vi "GetObserverList.vi"(8 "error in (no error)":errorcluster, 11 "Observable in":refnum<class "Observable.lvclass">) -> (0 "error out":errorcluster, 2 "ObserverClassName":string[](array[string]), 3 "Observable out":refnum<class "Observable.lvclass">)   [LabVIEW 2013, in "Observable.lvclass"]
uses:
  Observable.lvclass
  Observable.lvclass/Observable.ctl
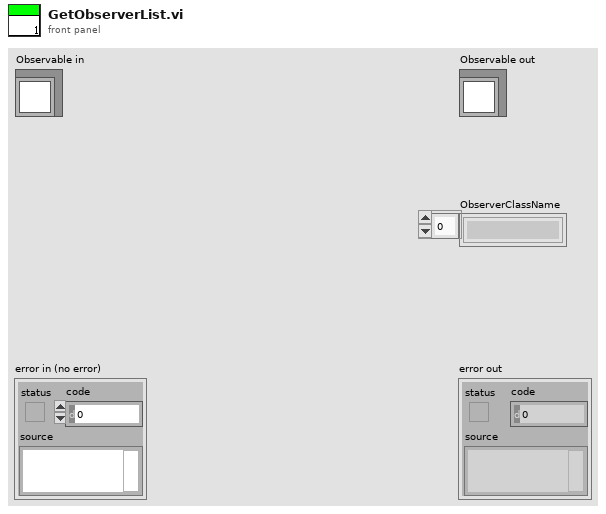
[diagram p1: front panel]
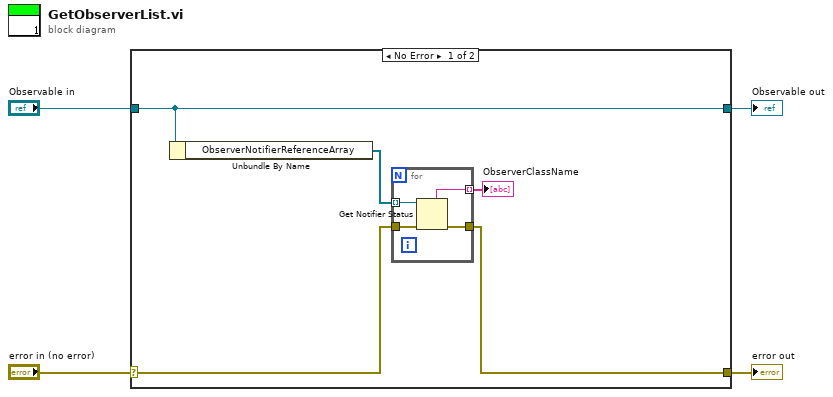
[diagram p0: block diagram]
diagram:
  n1 = case shown="No Error" "error in (no error)" {
    selector: "error in (no error)" -> [w7 w15]
    tunnel: [w6 w15] -> w3
    tunnel: [w9 w14] -> w1
    tunnel: "Observable in" -> [w9 w14]
    frame No Error {
      n2 = Unbundle By Name(w9) -> ("ObserverNotifierReferenceArray"=w8:refnum<notifier>[])
      n3 = for {
        tunnel: w8 -> [w13] mode=indexing
        tunnel: [w12] -> w5 mode=indexing
        tunnel: w7 -> [w11]
        tunnel: [w10] -> w6
        n4 = Get Notifier Status(notifier=w13, error in (no error)=w11) -> (notifier name=w12:string, error out=w10:errorcluster)  [unwired: 3 out]
      }
      "ObserverClassName" <- w5
    }
    frame Error {
    }
  }
  "error out" <- w3
  "Observable out" <- w1
